vi "Example 6017.vi"() -> ()   [LabVIEW 2024]
panel:
  out "Current mA":dbl
  in  "stop":bool
  out "Temp °C":dbl
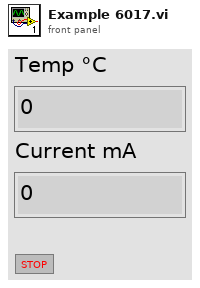
[diagram p1: front panel]
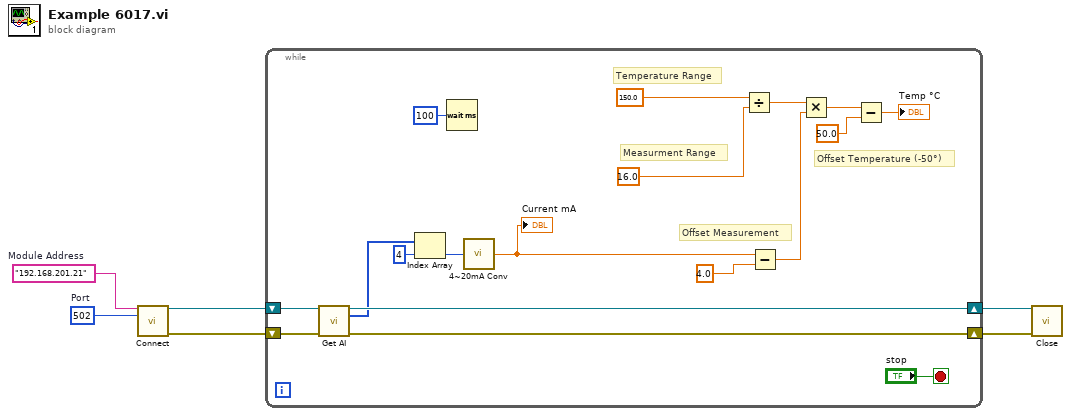
[diagram p0: block diagram]
diagram:
  w1 = u16 502  # Port
  w6 = "192.168.201.21"  # Module Address
  n1 = call "Connect.vi"("Module Address"=w6, "Port"=w1) -> ("Module Ref"=w5:refnum<class "Modbus Master.lvclass">, "error out"=w4:errorcluster)  [unwired: 12 in]
  n2 = while {
    shift-right: [w21] -> w3
    shift-left: w5 -> [w24]
    shift-right: [w22] -> w2
    shift-left: w4 -> [w23]
    stop <- "stop" stop-if-true
    # "Offset Temperature (-50°)"
    # "Offset Measurement"
    # "Measurment Range"
    # "Temperature Range"
    n3 = call "Get AI.vi"("Module Ref"=w24, "error in (no error)"=w23) -> ("Modbus master out"=w21:refnum<class "Modbus Master.lvclass">, "AI Measurment"=w20:u16[], "error out"=w22:errorcluster)  [unwired: 11 in]
    n4 = Index Array(array=w20, index=4) -> (element=w18:u16)
    n5 = Wait (ms)(milliseconds to wait=u32 100) -> ()  [unwired: 1 out]
    n6 = call "4~20mA Conv.vi"("Register Value"=w18) -> ("Current mA"=w14:dbl)
    "Current mA" <- w14
    n7 = Divide(x=150.0, y=16.0) -> (x/y=w15:dbl)
    n8 = Subtract(x=w14, y=4.0) -> (x-y=w12:dbl)
    n9 = Multiply(x=w15, y=w12) -> (x*y=w11:dbl)
    n10 = Subtract(x=w11, y=50.0) -> (x-y=→"Temp °C":dbl)
  }
  n11 = call "Close.vi"("Modbus master in"=w3, "error in (no error)"=w2) -> ()  [unwired: 13 in, 1 out]
